vi "ORS_AlazarDLLDigitalOut.vi"(8 "level":bool, 11 "error in (no error)":errorcluster) -> (0 "return code":i32, 1 "error out":errorcluster, 3 "path out":path=path "Z:/Software/AlazarTech/ATS-SDK/5.6.3/ATS9462-SDK/Dual Port Async/C/PostBuffer_Recommended/at_acquire/Release/at_acquire.dll")   [LabVIEW 2021]
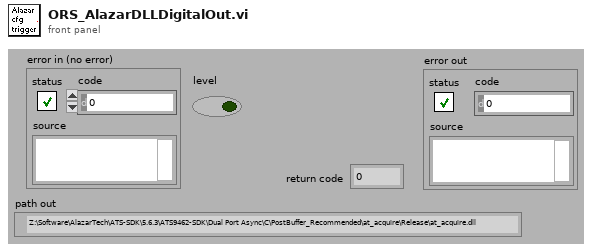
[diagram p1: front panel]
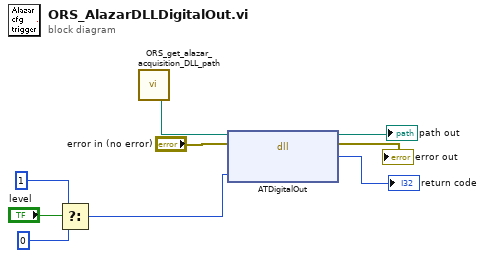
[diagram p0: block diagram]
diagram:
  n1 = Select(t=1, s="level", f=0) -> (s? t:f=w1:i32)
  n2 = call "ORS_get_alazar_acquisition_DLL_path.vi"() -> ("Alazar Acquisition DLL path"=w7:path)  [unwired: 10 in, 1 out]
  n3 = dll-call lib="Z:/Software/AlazarTech/ATS-SDK/5.6.3/ATS9462-SDK/Dual Port Async/C/PostBuffer_Recommended/at_acquire/Release/at_acquire.dll" fn="ATDigitalOut" ("at_acquire.dll:TestFunc")(path in=w7, error in="error in (no error)", "level"=w1) -> (path out=→"path out":path, error out=→"error out":errorcluster, "return type"=→"return code":i32)  [unwired: 2 in]
